vi "Get Pixel Formats.vi"(8 "error in (no error)":errorcluster, 11 "Camera in":refnum<class "Camera.lvclass">) -> (0 "error out":errorcluster, 2 "Pixel Formats":string[](array[string]), 3 "Camera":refnum<class "Camera.lvclass">)   [LabVIEW 2020, in "Camera.lvclass"]
uses:
  Camera.lvclass
  Camera.lvclass/Camera.ctl
  bin/gindustrialcam_32-1.dll
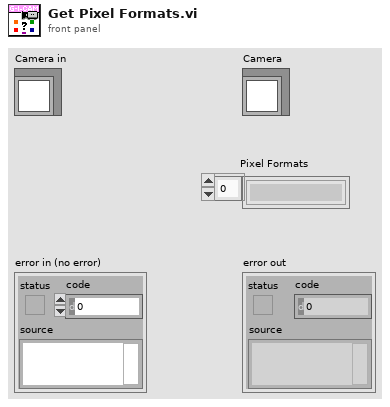
[diagram p1: front panel]
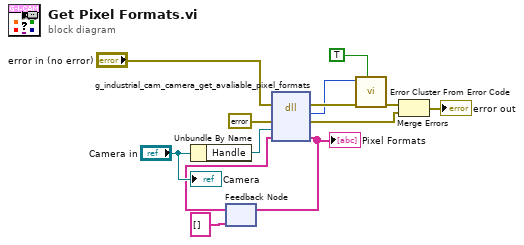
[diagram p0: block diagram]
diagram:
  n1 = Unbundle By Name("Camera in") -> ("Handle"=w1:refnum<data-value>)
  n2 = feedback #1(string[] []) -> (w3:string[])
  n3 = dll-call lib="C:/Workspace/SSDC/g-industrial-camera/LabVIEW/g_industrial_cam/bin/gindustrialcam_*-1.*" fn="g_industrial_cam_camera_get_avaliable_pixel_formats"(error in="error in (no error)", "err"=errorcluster {"status"=FALSE, "code"=0, "source"=""} ("error constant"), "edvr"=w1, "formats"=w3) -> (error out=w11:errorcluster, "Mg_Error"=w10:i32, "err"=w8:errorcluster, "formats"=w2:string[])  [unwired: 3 in, 1 out]
  "Pixel Formats" <- w2
  n4 = feedback-in #1(w2) -> ()
  n5 = call <vilib>:"Error Cluster From Error Code.vi"("show call chain? (False)"=TRUE, "error in (no error)"=w11, "error code (0)"=w10) -> ("error out"=w9:errorcluster)  [unwired: 6 in]
  n6 = Merge Errors(w9, w8) -> (→"error out":errorcluster)
  "Camera" <- "Camera in"
